vi "Table Color Clear Select.vi"(10 "Current Step ID":i32, 11 "Test Table":refnum<vi>) -> ()   [LabVIEW 2018]
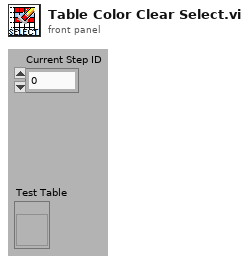
[diagram p1: front panel]
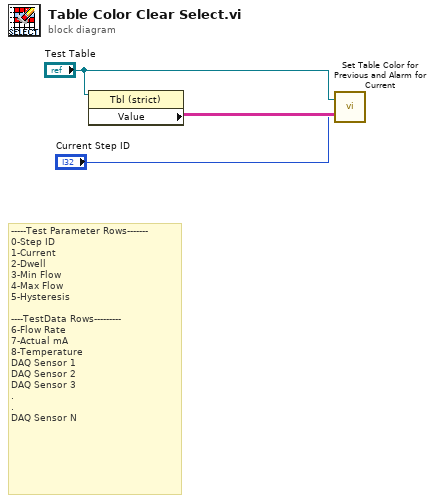
[diagram p0: block diagram]
diagram:
  # "-----Test Parameter Rows-------\n0-Step ID\n1-Current\n2-Dwell\n3-Min Flow\n4-Max Flow\n5-Hysteresis\n\n----TestData Rows---------\n6-Flow Rate\n7-Actual mA\n8-Temperature\nDAQ Sensor 1\nDAQ Sensor 2\nDAQ Sensor 3\n.\n.\nDAQ Sensor N"
  n1 = property class="Tbl (strict)"(reference="Test Table") -> ("Value"=w3:string[][])  [unwired: 1 in, 2 out]
  n2 = call "Set Table Color for Previous and Alarm for Current.vi"("Test Table"="Test Table", "Previous Step ID"="Current Step ID", "Value"=w3) -> ()  [unwired: 13 in]
